vi "Algo_FCI_Overlay.vi"(6 "Overlay cluster out":T4={"Lip Level"={"Lip Gap Overlay ROI 1"=[], "Lip Gap ROi Overlay 2"=[]}, "EON outer width cluster out"={"Search Lines out"=[], "Start End Points\nIndex"=0.0, "Perpendicular lines to ROI\ncluster out"=[{{"X"=55.0, "Y"=48.0}, {"X"=263.0, "Y"=104.0}}, {{"X"=53.0, "Y"=53.0}, {"X"=262.0, "Y"=109.0}}, {{"X"=52.0, "Y"=58.0}, {"X"=261.0, "Y"=113.0}}, {{"X"=51.0, "Y"=62.0}, {"X"=259.0, "Y"=118.0}}, {{"X"=49.0, "Y"=67.0}, {"X"=258.0, "Y"=123.0}}, {{"X"=48.0, "Y"=72.0}, {"X"=257.0, "Y"=128.0}}, {{"X"=47.0, "Y"=77.0}, {"X"=255.0, "Y"=133.0}}, {{"X"=46.0, "Y"=82.0}, {"X"=254.0, "Y"=138.0}}, {{"X"=44.0, "Y"=87.0}, {"X"=253.0, "Y"=142.0}}, {{"X"=43.0, "Y"=91.0}, {"X"=252.0, "Y"=147.0}}, {{"X"=42.0, "Y"=96.0}, {"X"=250.0, "Y"=152.0}}]}, "Box width cluster out"={"Start Point array out"=[], "End point array out"=[], "Last Edges location array out"=[], "Search lines location\narray out"=[], "Array Index"=0.0}, "Lip Gap cluster out"={"Perpendicular Lines"=[{{"X"=55.0, "Y"=48.0}, {"X"=263.0, "Y"=104.0}}, {{"X"=53.0, "Y"=53.0}, {"X"=262.0, "Y"=109.0}}, {{"X"=52.0, "Y"=58.0}, {"X"=261.0, "Y"=113.0}}, {{"X"=51.0, "Y"=62.0}, {"X"=259.0, "Y"=118.0}}, {{"X"=49.0, "Y"=67.0}, {"X"=258.0, "Y"=123.0}}, {{"X"=48.0, "Y"=72.0}, {"X"=257.0, "Y"=128.0}}, {{"X"=47.0, "Y"=77.0}, {"X"=255.0, "Y"=133.0}}, {{"X"=46.0, "Y"=82.0}, {"X"=254.0, "Y"=138.0}}, {{"X"=44.0, "Y"=87.0}, {"X"=253.0, "Y"=142.0}}, {{"X"=43.0, "Y"=91.0}, {"X"=252.0, "Y"=147.0}}, {{"X"=42.0, "Y"=96.0}, {"X"=250.0, "Y"=152.0}}], "Search Lines"=[]}, "102 Lip Gap cluster out"={"102 Lip Gap ROI out"={"Global Rectangle"=[], "Contours"=[]}, "102 Lip gap overlay\npoints array"=[]}, "Lip outer width cluster out"={"Start Point"={"X"=0.0, "Y"=0.0}, "End Point"={"X"=0.0, "Y"=0.0}, "Perpendicular Lines"=[{{"X"=55.0, "Y"=48.0}, {"X"=263.0, "Y"=104.0}}, {{"X"=53.0, "Y"=53.0}, {"X"=262.0, "Y"=109.0}}, {{"X"=52.0, "Y"=58.0}, {"X"=261.0, "Y"=113.0}}, {{"X"=51.0, "Y"=62.0}, {"X"=259.0, "Y"=118.0}}, {{"X"=49.0, "Y"=67.0}, {"X"=258.0, "Y"=123.0}}, {{"X"=48.0, "Y"=72.0}, {"X"=257.0, "Y"=128.0}}, {{"X"=47.0, "Y"=77.0}, {"X"=255.0, "Y"=133.0}}, {{"X"=46.0, "Y"=82.0}, {"X"=254.0, "Y"=138.0}}, {{"X"=44.0, "Y"=87.0}, {"X"=253.0, "Y"=142.0}}, {{"X"=43.0, "Y"=91.0}, {"X"=252.0, "Y"=147.0}}, {{"X"=42.0, "Y"=96.0}, {"X"=250.0, "Y"=152.0}}]}, "Lip symmetry out"={"Lip symmetry points array 2"=[], "Lip Symmetry Points array 1"=[]}} {"Lip symmetry out"."Lip Symmetry Points array 1"."Y" format="%.2f"; "Lip symmetry out"."Lip Symmetry Points array 1"."X" format="%.2f"; "Lip outer width cluster out"."Perpendicular Lines"."?"."Y" format="%.2f"; "Lip outer width cluster out"."Perpendicular Lines"."?"."X" format="%.2f"; "Lip outer width cluster out"."Perpendicular Lines"."?"."Y" format="%.2f"; "Lip outer width cluster out"."Perpendicular Lines"."?"."X" format="%.2f"; "102 Lip Gap cluster out"."102 Lip Gap ROI out"."Contours"."Type" items=["No Selection", "Point", "Line", "Rectangle", "Oval", "Polygon", "Freehand Region", "Annulus", "Unused2", "Unused3", "Broken Line", "Freehand Line", "Rotated Rectangle"]; "Lip Gap cluster out"."Search Lines"."Edge Info"."Distance (Real-World)" format="%.2f"; "Lip Gap cluster out"."Search Lines"."Edge Info"."Location (Real-World)"."Y" format="%.2g"; "Lip Gap cluster out"."Search Lines"."Edge Info"."Location (Real-World)"."X" format="%.2f"; "Lip Gap cluster out"."Search Lines"."Edge Info"."Noise" format="%.2f"; "Lip Gap cluster out"."Search Lines"."Edge Info"."Location (Pixel)"."Y" format="%.2g"; "Lip Gap cluster out"."Search Lines"."Edge Info"."Location (Pixel)"."X" format="%.2f"; "Lip Gap cluster out"."Search Lines"."Edge Info"."Strength" format="%.2f"; "Lip Gap cluster out"."Search Lines"."Edge Info"."Distance (Pixel)" format="%.2f"; "Lip Gap cluster out"."Perpendicular Lines"."?"."Y" format="%.2f"; "Lip Gap cluster out"."Perpendicular Lines"."?"."X" format="%.2f"; "Lip Gap cluster out"."Perpendicular Lines"."?"."Y" format="%.2f"; "Lip Gap cluster out"."Perpendicular Lines"."?"."X" format="%.2f"; "EON outer width cluster out"."Perpendicular lines to ROI\ncluster out"."?"."Y" format="%.2f"; "EON outer width cluster out"."Perpendicular lines to ROI\ncluster out"."?"."X" format="%.2f"; "EON outer width cluster out"."Perpendicular lines to ROI\ncluster out"."?"."Y" format="%.2f"; "EON outer width cluster out"."Perpendicular lines to ROI\ncluster out"."?"."X" format="%.2f"; "EON outer width cluster out"."Search Lines out"."Edge Info"."Distance (Real-World)" format="%.2f"; "EON outer width cluster out"."Search Lines out"."Edge Info"."Location (Real-World)"."Y" format="%.2g"; "EON outer width cluster out"."Search Lines out"."Edge Info"."Location (Real-World)"."X" format="%.2f"; "EON outer width cluster out"."Search Lines out"."Edge Info"."Noise" format="%.2f"; "EON outer width cluster out"."Search Lines out"."Edge Info"."Location (Pixel)"."Y" format="%.2g"; "EON outer width cluster out"."Search Lines out"."Edge Info"."Location (Pixel)"."X" format="%.2f"; "EON outer width cluster out"."Search Lines out"."Edge Info"."Strength" format="%.2f"; "EON outer width cluster out"."Search Lines out"."Edge Info"."Distance (Pixel)" format="%.2f"; "Lip Level"."Lip Gap Overlay ROI 1"."Y" format="%.2f"; "Lip Level"."Lip Gap Overlay ROI 1"."X" format="%.2f"}, 7 "Pass?":bool, 8 "error in (no error)":errorcluster, 9 "Image in":T5, 10 "Algo Type":T6=enum."Linear", 11 "Enabled?":bool) -> (0 "error out":errorcluster)   [LabVIEW 2015, in "Algorithm.lvclass"]
uses:
  FrameworkOverrides/Algorithm.lvclass
  Controls/Algo_Type.ctl
  <vilib>/vision/Image Controls.llb/IMAQ Image.ctl
  <vilib>/vision/Measure.llb/Search Line.ctl
  <vilib>/vision/Measure.llb/Edge New.ctl
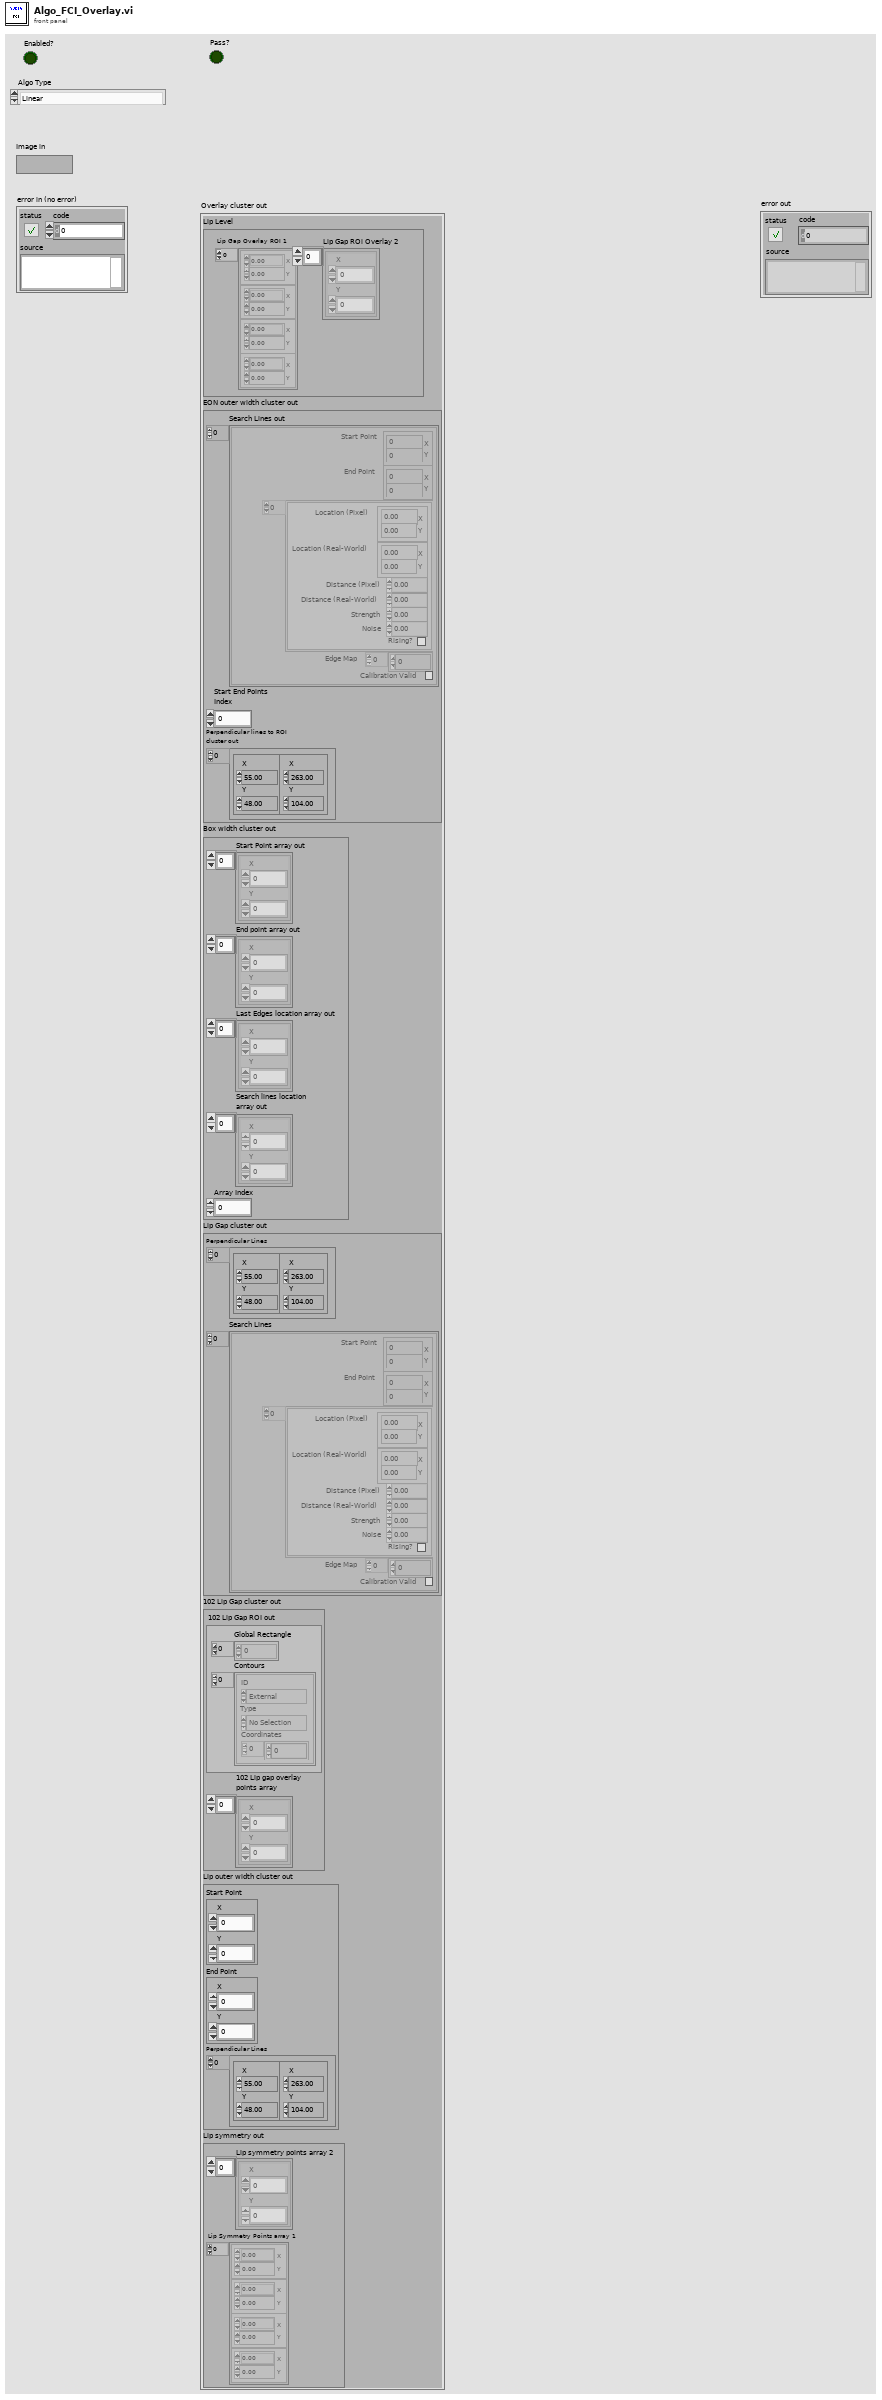
[diagram p1: front panel]
types:
  T1 = typedef "Search Line.ctl" = cluster{"Start Point":cluster{"X":sgl, "Y":sgl}, "End Point":cluster{"X":sgl, "Y":sgl}, "Edge Info":T2[], "Edge Map":dbl[], "Calibration Valid":bool}
  T2 = typedef "Edge New.ctl" = cluster{"Location (Pixel)":cluster{"X":sgl, "Y":sgl}, "Location (Real-World)":cluster{"X":sgl, "Y":sgl}, "Distance (Pixel)":dbl, "Distance (Real-World)":dbl, "Strength":dbl, "Noise":dbl, "Rising?":bool}
  T3 = typedef "ROI Descriptor" = cluster{"Global Rectangle":i32[], "Contours":cluster{"ID":enum32{"External", "Internal"}, "Type":u32, "Coordinates":i32[]}[]}
  T4 = cluster{"Lip Level":cluster{"Lip Gap Overlay ROI 1":cluster{"X":sgl, "Y":sgl}[], "Lip Gap ROi Overlay 2":cluster{"X":sgl, "Y":sgl}[]}, "EON outer width cluster out":cluster{"Search Lines out":T1[], "Start End Points\nIndex":dbl, "Perpendicular lines to ROI\ncluster out":cluster{cluster{"X":sgl, "Y":sgl}, cluster{"X":sgl, "Y":sgl}}[]}, "Box width cluster out":cluster{"Start Point array out":cluster{"X":sgl, "Y":sgl}[], "End point array out":cluster{"X":sgl, "Y":sgl}[], "Last Edges location array out":cluster{"X":sgl, "Y":sgl}[], "Search lines location\narray out":cluster{"X":sgl, "Y":sgl}[], "Array Index":dbl}, "Lip Gap cluster out":cluster{"Perpendicular Lines":cluster{cluster{"X":sgl, "Y":sgl}, cluster{"X":sgl, "Y":sgl}}[], "Search Lines":T1[]}, "102 Lip Gap cluster out":cluster{"102 Lip Gap ROI out":T3, "102 Lip gap overlay\npoints array":cluster{"X":sgl, "Y":sgl}[]}, "Lip outer width cluster out":cluster{"Start Point":cluster{"X":sgl, "Y":sgl}, "End Point":cluster{"X":sgl, "Y":sgl}, "Perpendicular Lines":cluster{cluster{"X":sgl, "Y":sgl}, cluster{"X":sgl, "Y":sgl}}[]}, "Lip symmetry out":cluster{"Lip symmetry points array 2":cluster{"X":sgl, "Y":sgl}[], "Lip Symmetry Points array 1":cluster{"X":sgl, "Y":sgl}[]}}
  T5 = typedef "IMAQ Image.ctl" = refnum<image>
  T6 = typedef "Algorithm.lvclass/Algo_Type.ctl" = enum16{"Lancing Presence", "Pitch", "Circlular_Dia", "LipGap", "Angle", "BarbHeight", "102 EON Presence", "102 Lipgap", "Lip Symmetry", "Lip Level", "Box Width", "Lip Outer Width", "EON Width", "EON Presence", "Lipgap FCI", "Linear", "Projected Distance_Type_1", " Projected Distance_Type_2", "Projected Distance_Type_3", "AET", "AET Min", "TT_Width", "Lancing", "WND", "Linear_Lenght1", "Linear_Lenght2", "Side_E", "Side_E1", "Top_E", "Edge Distance", "Side Vertical Minimum"}
  T7 = cluster{cluster{"X":sgl, "Y":sgl}, cluster{"X":sgl, "Y":sgl}}[]
  T8 = cluster{"Start Point":cluster{"X":sgl, "Y":sgl}, cluster{"X":sgl, "Y":sgl}}
  T9 = cluster{cluster{"X":sgl, "Y":sgl}, "End Point":cluster{"X":sgl, "Y":sgl}}
  T10 = cluster{"Start Point":cluster{"X":sgl, "Y":sgl}, "Location (Pixel)":cluster{"X":sgl, "Y":sgl}}
  T11 = cluster{"Location (Pixel)":cluster{"X":sgl, "Y":sgl}, "End Point":cluster{"X":sgl, "Y":sgl}}
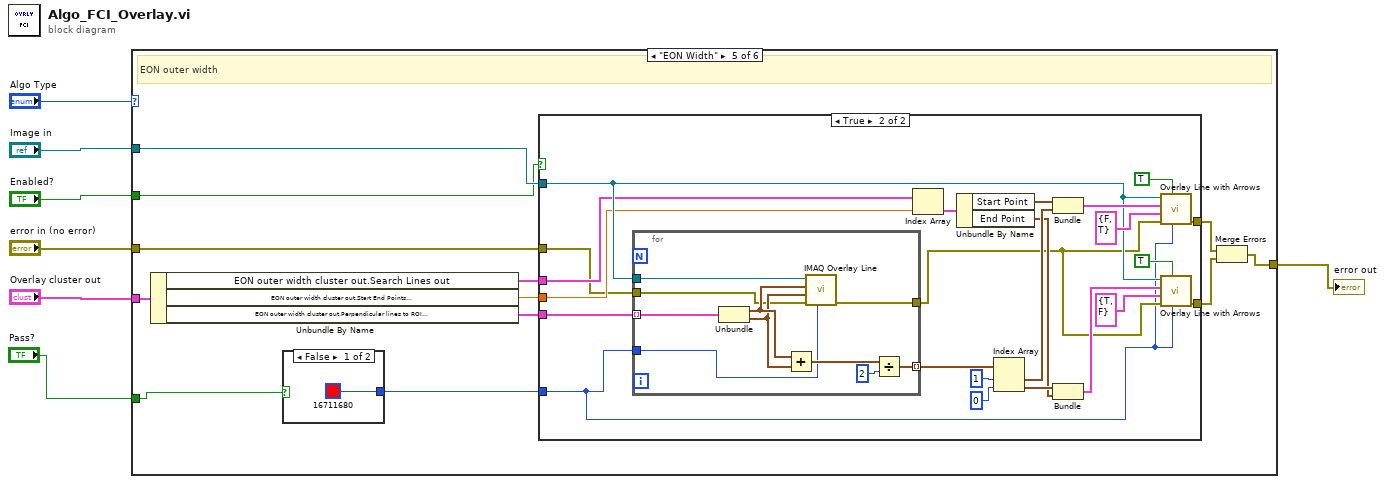
[diagram p0: block diagram]
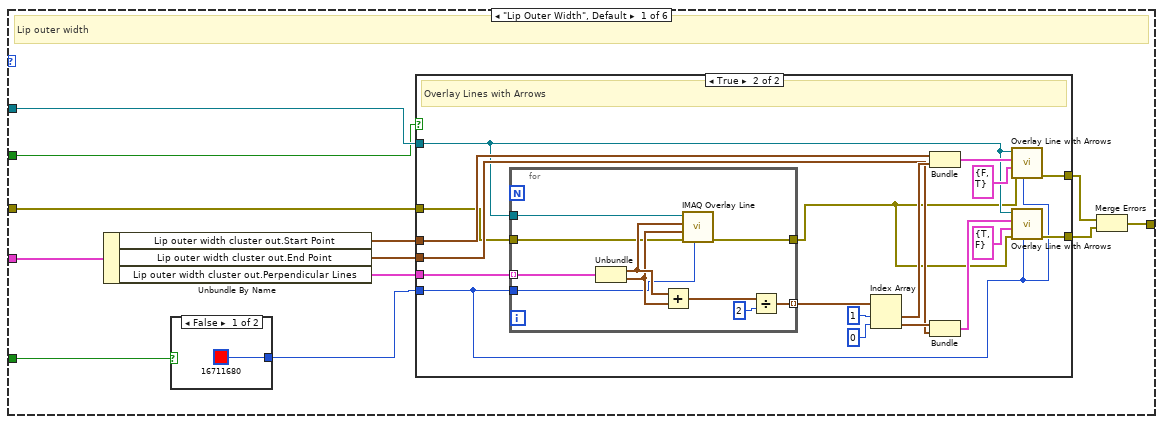
[diagram p2: hidden frame]
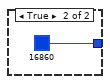
[diagram p3: hidden frame]
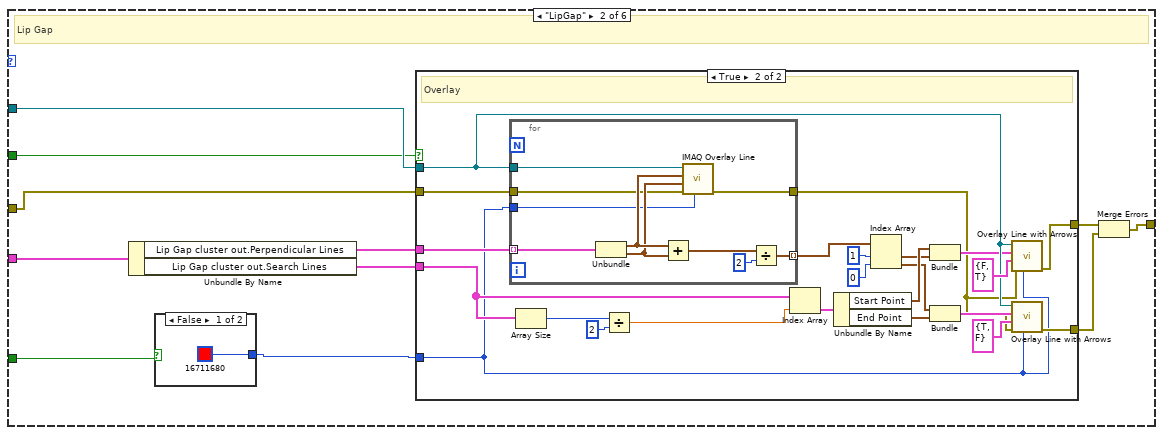
[diagram p5: hidden frame]
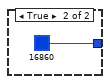
[diagram p6: hidden frame]
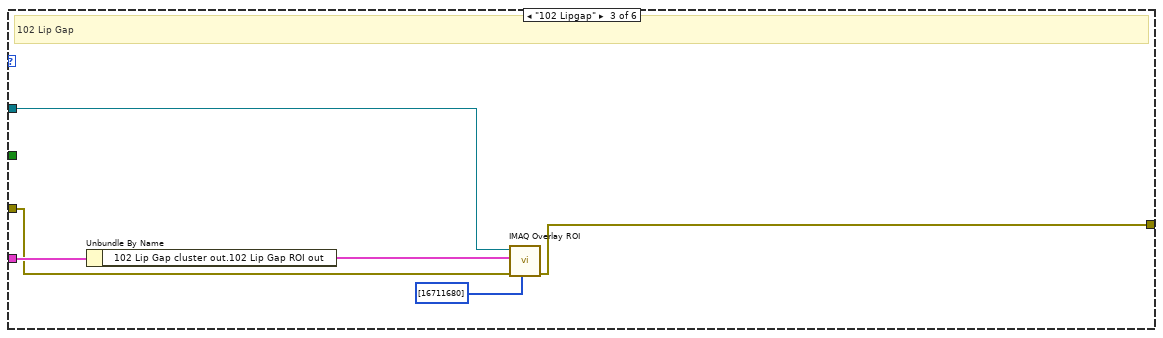
[diagram p8: hidden frame]
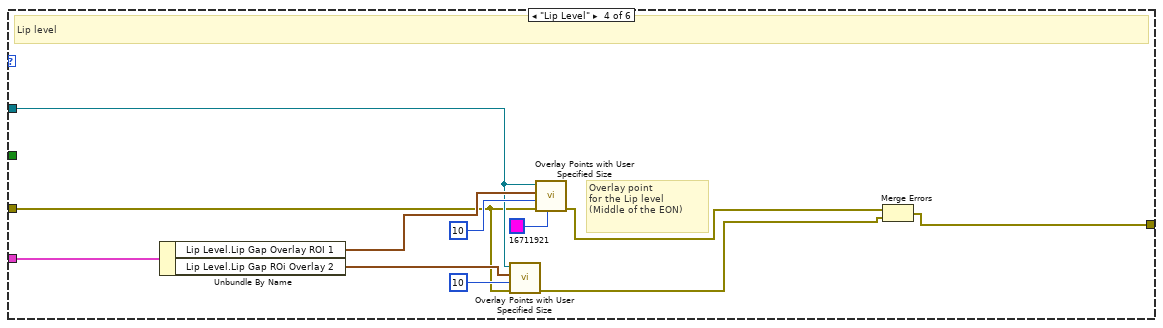
[diagram p9: hidden frame]
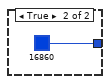
[diagram p10: hidden frame]
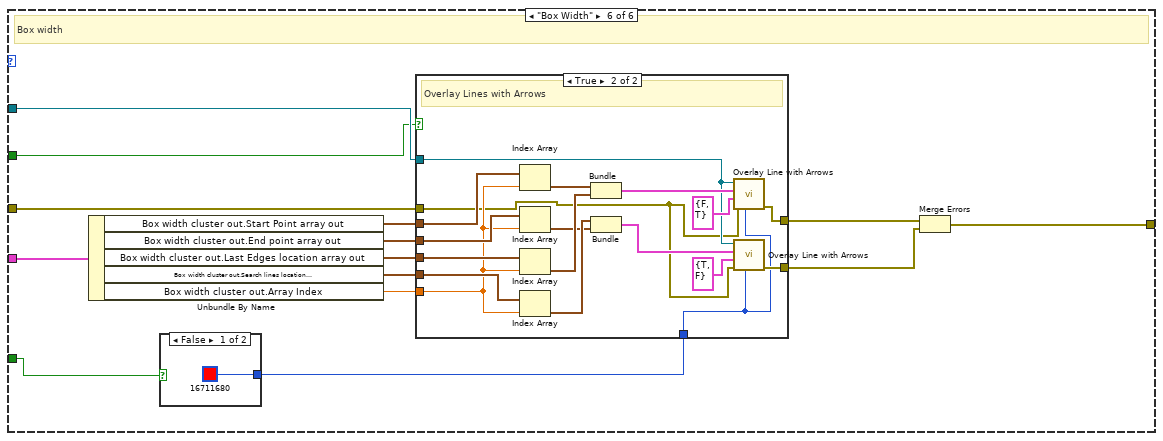
[diagram p12: hidden frame]
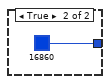
[diagram p13: hidden frame]
diagram:
  n1 = case shown="\"EON Width\"" "Algo Type" {
    tunnel: "Overlay cluster out" -> [w19 w61 w102 w111 w125 w176]
    tunnel: "Image in" -> [w15 w58 w100 w108 w126 w171]
    tunnel: "error in (no error)" -> [w13 w56 w99 w107 w120 w168]
    tunnel: "Enabled?" -> [w14 w57 _ _ w121 w169]
    tunnel: [w10 w53 w98 w104 w117 w165] -> w2
    tunnel: "Pass?" -> [w9 w52 _ _ w116 w164]
    frame "Lip Outer Width", Default {
      # "Lip outer width"
      n2 = Unbundle By Name(w19) -> ("Lip outer width cluster out.Start Point"=w17:cluster{"X":sgl, "Y":sgl}, "Lip outer width cluster out.End Point"=w16:cluster{"X":sgl, "Y":sgl}, "Lip outer width cluster out.Perpendicular Lines"=w18:T7)
      n3 = case shown="False" w9 {
        tunnel: [u32 16711680 u32 16860] -> w8
        frame False {
        }
        frame True {
        }
      }
      n4 = case shown="True" w14 {
        tunnel: w18 -> [_ w40]
        tunnel: w17 -> [_ w38]
        tunnel: w16 -> [_ w33]
        tunnel: w15 -> [_ w28]
        tunnel: w13 -> [w22 w27]
        tunnel: [w22 w25] -> w12
        tunnel: [w22 w24] -> w11
        tunnel: w8 -> [_ w23]
        frame False {
        }
        frame True {
          # "Overlay Lines with Arrows"
          n5 = for {
            tunnel: w40 -> [w50] mode=indexing
            tunnel: w28 -> [w49]
            tunnel: [w44] -> w39 mode=indexing
            tunnel: w27 -> [w43]
            tunnel: [w42] -> w26
            tunnel: w23 -> [w41]
            n6 = Unbundle(w50) -> (w48:cluster{"X":sgl, "Y":sgl}, w47:cluster{"X":sgl, "Y":sgl})
            n7 = Add(x=w48, y=w47) -> (x+y=w46:cluster{"X":sgl, "Y":sgl})
            n8 = call "IMAQ Overlay Line"("Color"=w41, "error in (no error)"=w43, "End Point"=w47, "Start Point"=w48, "Image"=w49) -> ("error out"=w42:errorcluster)  [unwired: 5 in, 1 out]
            n9 = Divide(x=w46, y=2) -> (x/y=w44:cluster{"X":sgl, "Y":sgl})
          }
          n10 = Index Array(array=w39, index #1=1 ("index"), index #2=0 ("index")) -> (element #1=w36:cluster{"X":sgl, "Y":sgl}, element #2=w34:cluster{"X":sgl, "Y":sgl})
          n11 = Bundle("Start Point"=w38, w36) -> (w32:T8)  [unwired: 1 in]
          n12 = Bundle(w34, "End Point"=w33) -> (w30:T9)  [unwired: 1 in]
          n13 = call <vilib>:"Overlay Line with Arrows.vi"("Color"=w23, "error in (no error)"=w26, "Arrows"=cluster{"Start point":bool, "End point":bool} {"Start point"=FALSE, "End point"=TRUE}, "Line Coordinates"=w32, "Image In"=w28) -> ("error out"=w25:errorcluster)  [unwired: 5 in, 1 out]
          n14 = call <vilib>:"Overlay Line with Arrows.vi"("Color"=w23, "error in (no error)"=w26, "Arrows"=cluster{"Start point":bool, "End point":bool} {"Start point"=TRUE, "End point"=FALSE}, "Line Coordinates"=w30, "Image In"=w28) -> ("error out"=w24:errorcluster)  [unwired: 5 in, 1 out]
        }
      }
      n15 = Merge Errors(w12, w11) -> (w10:errorcluster)
    }
    frame "LipGap" {
      # "Lip Gap"
      n16 = Unbundle By Name(w61) -> ("Lip Gap cluster out.Perpendicular Lines"=w60:T7, "Lip Gap cluster out.Search Lines"=w59:T1[])
      n17 = case shown="False" w52 {
        tunnel: [u32 16711680 u32 16860] -> w51
        frame False {
        }
        frame True {
        }
      }
      n18 = case shown="True" w57 {
        tunnel: w60 -> [_ w87]
        tunnel: w58 -> [_ w79]
        tunnel: w59 -> [_ w84]
        tunnel: w56 -> [w64 w69]
        tunnel: [w64 w68] -> w55
        tunnel: [w64 w66] -> w54
        tunnel: w51 -> [_ w65]
        frame False {
        }
        frame True {
          # "Overlay"
          n19 = for {
            tunnel: w87 -> [w97] mode=indexing
            tunnel: w79 -> [w96]
            tunnel: [w91] -> w78 mode=indexing
            tunnel: w69 -> [w90]
            tunnel: [w89] -> w67
            tunnel: w65 -> [w88]
            n20 = Unbundle(w97) -> (w95:cluster{"X":sgl, "Y":sgl}, w94:cluster{"X":sgl, "Y":sgl})
            n21 = Add(x=w95, y=w94) -> (x+y=w93:cluster{"X":sgl, "Y":sgl})
            n22 = call "IMAQ Overlay Line"("Color"=w88, "error in (no error)"=w90, "End Point"=w94, "Start Point"=w95, "Image"=w96) -> ("error out"=w89:errorcluster)  [unwired: 5 in, 1 out]
            n23 = Divide(x=w93, y=2) -> (x/y=w91:cluster{"X":sgl, "Y":sgl})
          }
          n24 = Array Size(array=w84) -> (size(s)=w86:i32)
          n25 = Divide(x=w86, y=2) -> (x/y=w83:dbl)
          n26 = Index Array(array=w84, index=w83) -> (element=w82:T1)
          n27 = Unbundle By Name(w82) -> ("Start Point"=w77:cluster{"X":sgl, "Y":sgl}, "End Point"=w74:cluster{"X":sgl, "Y":sgl})
          n28 = Index Array(array=w78, index #1=1 ("index"), index #2=0 ("index")) -> (element #1=w76:cluster{"X":sgl, "Y":sgl}, element #2=w75:cluster{"X":sgl, "Y":sgl})
          n29 = Bundle("Start Point"=w77, w76) -> (w73:T8)  [unwired: 1 in]
          n30 = Bundle(w75, "End Point"=w74) -> (w72:T9)  [unwired: 1 in]
          n31 = call <vilib>:"Overlay Line with Arrows.vi"("Color"=w65, "error in (no error)"=w67, "Arrows"=cluster{"Start point":bool, "End point":bool} {"Start point"=FALSE, "End point"=TRUE}, "Line Coordinates"=w73, "Image In"=w79) -> ("error out"=w68:errorcluster)  [unwired: 5 in, 1 out]
          n32 = call <vilib>:"Overlay Line with Arrows.vi"("Color"=w65, "error in (no error)"=w67, "Arrows"=cluster{"Start point":bool, "End point":bool} {"Start point"=TRUE, "End point"=FALSE}, "Line Coordinates"=w72, "Image In"=w79) -> ("error out"=w66:errorcluster)  [unwired: 5 in, 1 out]
        }
      }
      n33 = Merge Errors(w55, w54) -> (w53:errorcluster)
    }
    frame "102 Lipgap" {
      # "102 Lip Gap"
      n34 = Unbundle By Name(w102) -> ("102 Lip Gap cluster out.102 Lip Gap ROI out"=w101:T3)
      n35 = call "IMAQ Overlay ROI"("Colors (Green)"=u32[] [16711680], "error in (no error)"=w99, "ROI Descriptor"=w101, "Image"=w100) -> ("error out"=w98:errorcluster)  [unwired: 6 in, 1 out]
    }
    frame "Lip Level" {
      # "Overlay point \nfor the Lip level\n(Middle of the EON)"
      # "Lip level"
      n36 = Unbundle By Name(w111) -> ("Lip Level.Lip Gap Overlay ROI 1"=w110:cluster{"X":sgl, "Y":sgl}[], "Lip Level.Lip Gap ROi Overlay 2"=w109:cluster{"X":sgl, "Y":sgl}[])
      n37 = call "Overlay Points with User Specified Size.vi"("error in"=w107, "Point Diameter (5)"=u32 10, "Points"=w109, "Image In"=w108) -> ("error out"=w105:errorcluster)  [unwired: 6 in, 1 out]
      n38 = call "Overlay Points with User Specified Size.vi"("Color"=u32 16711921, "error in"=w107, "Point Diameter (5)"=u32 10, "Points"=w110, "Image In"=w108) -> ("error out"=w106:errorcluster)  [unwired: 5 in, 1 out]
      n39 = Merge Errors(w106, w105) -> (w104:errorcluster)
    }
    frame "EON Width" {
      # "EON outer width"
      n40 = Unbundle By Name(w125) -> ("EON outer width cluster out.Search Lines out"=w124:T1[], "EON outer width cluster out.Start End Points\nIndex"=w123:dbl, "EON outer width cluster out.Perpendicular lines to ROI\ncluster out"=w122:T7)
      n41 = case shown="False" w116 {
        tunnel: [u32 16711680 u32 16860] -> w115
        frame False {
        }
        frame True {
        }
      }
      n42 = case shown="True" w121 {
        tunnel: w122 -> [_ w146]
        tunnel: w126 -> [_ w140]
        tunnel: w124 -> [_ w139]
        tunnel: w123 -> [_ w137]
        tunnel: w120 -> [w129 w134]
        tunnel: [w129 w132] -> w119
        tunnel: [w129 w131] -> w118
        tunnel: w115 -> [_ w130]
        frame False {
        }
        frame True {
          n43 = for {
            tunnel: w146 -> [w162] mode=indexing
            tunnel: w140 -> [w161]
            tunnel: [w156] -> w145 mode=indexing
            tunnel: w134 -> [w155]
            tunnel: [w154] -> w133
            tunnel: w130 -> [w153]
            n44 = Unbundle(w162) -> (w160:cluster{"X":sgl, "Y":sgl}, w159:cluster{"X":sgl, "Y":sgl})
            n45 = Add(x=w160, y=w159) -> (x+y=w158:cluster{"X":sgl, "Y":sgl})
            n46 = call "IMAQ Overlay Line"("Color"=w153, "error in (no error)"=w155, "End Point"=w159, "Start Point"=w160, "Image"=w161) -> ("error out"=w154:errorcluster)  [unwired: 5 in, 1 out]
            n47 = Divide(x=w158, y=2) -> (x/y=w156:cluster{"X":sgl, "Y":sgl})
          }
          n48 = Index Array(array=w139, index=w137) -> (element=w138:T1)
          n49 = Unbundle By Name(w138) -> ("Start Point"=w135:cluster{"X":sgl, "Y":sgl}, "End Point"=w136:cluster{"X":sgl, "Y":sgl})
          n50 = Index Array(array=w145, index #1=1 ("index"), index #2=0 ("index")) -> (element #1=w144:cluster{"X":sgl, "Y":sgl}, element #2=w143:cluster{"X":sgl, "Y":sgl})
          n51 = Bundle("Start Point"=w135, w144) -> (w152:T8)  [unwired: 1 in]
          n52 = Bundle(w143, "End Point"=w136) -> (w147:T9)  [unwired: 1 in]
          n53 = call <vilib>:"Overlay Line with Arrows.vi"("Color"=w130, "Draw line?"=TRUE, "error in (no error)"=w133, "Arrows"=cluster{"Start point":bool, "End point":bool} {"Start point"=FALSE, "End point"=TRUE}, "Line Coordinates"=w152, "Image In"=w140) -> ("error out"=w132:errorcluster)  [unwired: 4 in, 1 out]
          n54 = call <vilib>:"Overlay Line with Arrows.vi"("Color"=w130, "Draw line?"=TRUE, "error in (no error)"=w133, "Arrows"=cluster{"Start point":bool, "End point":bool} {"Start point"=TRUE, "End point"=FALSE}, "Line Coordinates"=w147, "Image In"=w140) -> ("error out"=w131:errorcluster)  [unwired: 4 in, 1 out]
        }
      }
      n55 = Merge Errors(w119, w118) -> (w117:errorcluster)
    }
    frame "Box Width" {
      # "Box width"
      n56 = Unbundle By Name(w176) -> ("Box width cluster out.Start Point array out"=w175:cluster{"X":sgl, "Y":sgl}[], "Box width cluster out.End point array out"=w174:cluster{"X":sgl, "Y":sgl}[], "Box width cluster out.Last Edges location array out"=w173:cluster{"X":sgl, "Y":sgl}[], "Box width cluster out.Search lines location\narray out"=w172:cluster{"X":sgl, "Y":sgl}[], "Box width cluster out.Array Index"=w170:dbl)
      n57 = case shown="False" w164 {
        tunnel: [u32 16711680 u32 16860] -> w163
        frame False {
        }
        frame True {
        }
      }
      n58 = case shown="True" w169 {
        tunnel: w173 -> [_ w197]
        tunnel: w172 -> [_ w196]
        tunnel: w175 -> [_ w195]
        tunnel: w174 -> [_ w194]
        tunnel: w170 -> [_ w193]
        tunnel: w171 -> [_ w184]
        tunnel: w168 -> [w179 w183]
        tunnel: [w179 w182] -> w167
        tunnel: [w179 w181] -> w166
        tunnel: w163 -> [_ w180]
        frame False {
        }
        frame True {
          # "Overlay Lines with Arrows"
          n59 = Index Array(array=w195, index=w193) -> (element=w188:cluster{"X":sgl, "Y":sgl})
          n60 = Index Array(array=w194, index=w193) -> (element=w185:cluster{"X":sgl, "Y":sgl})
          n61 = Index Array(array=w197, index=w193) -> (element=w187:cluster{"X":sgl, "Y":sgl})
          n62 = Index Array(array=w196, index=w193) -> (element=w186:cluster{"X":sgl, "Y":sgl})
          n63 = Bundle("Start Point"=w188, "Location (Pixel)"=w187) -> (w189:T10)  [unwired: 1 in]
          n64 = Bundle("Location (Pixel)"=w186, "End Point"=w185) -> (w190:T11)  [unwired: 1 in]
          n65 = call <vilib>:"Overlay Line with Arrows.vi"("Color"=w180, "error in (no error)"=w183, "Arrows"=cluster{"Start point":bool, "End point":bool} {"Start point"=FALSE, "End point"=TRUE}, "Line Coordinates"=w189, "Image In"=w184) -> ("error out"=w182:errorcluster)  [unwired: 5 in, 1 out]
          n66 = call <vilib>:"Overlay Line with Arrows.vi"("Color"=w180, "error in (no error)"=w183, "Arrows"=cluster{"Start point":bool, "End point":bool} {"Start point"=TRUE, "End point"=FALSE}, "Line Coordinates"=w190, "Image In"=w184) -> ("error out"=w181:errorcluster)  [unwired: 5 in, 1 out]
        }
      }
      n67 = Merge Errors(w167, w166) -> (w165:errorcluster)
    }
  }
  "error out" <- w2
